vi "SetCaptureFrames.vi"(8 "error in (no error)":errorcluster, 10 "Setting.FramesToCapture":i32, 11 "Camera_Prime95B in":refnum<class "Camera_Prime95B.lvclass">) -> (0 "error out":errorcluster, 3 "Camera_Prime95B out":refnum<class "Camera_Prime95B.lvclass">)   [LabVIEW 2020, in "Camera_Prime95B.lvlib" / "Camera_Prime95B.lvclass"]
uses:
  Camera_Prime95B.lvclass
  Camera_Prime95B.lvclass/Camera_Prime95B.ctl
  E:/Development/DevHardSoftware/MMicroscopyAF/Model/Real Hardware/Camera_Prime95B/Camera_Prime95B/Dependencies/PVCamNET.dll
  Dependencies/PVCamNET.dll
  HAL Layer/Component/Camera/Camera/Camera.lvclass
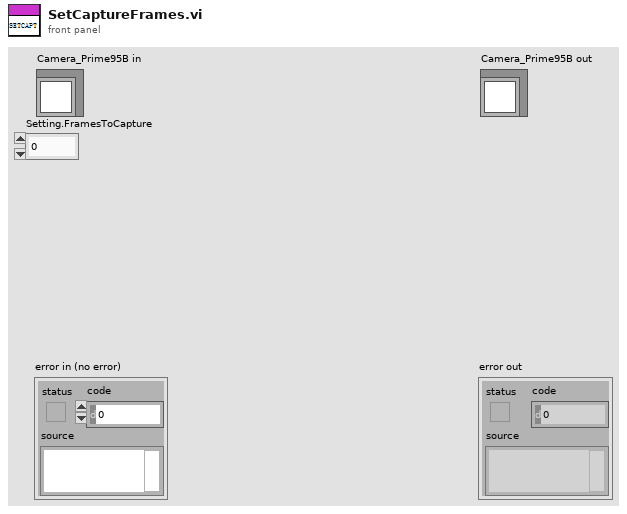
[diagram p1: front panel]
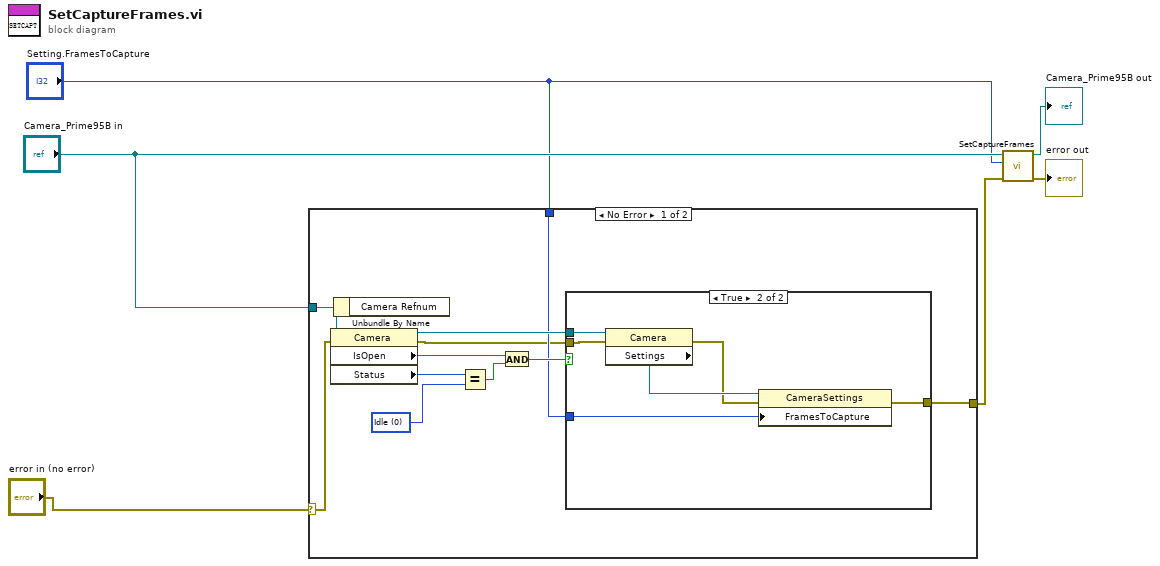
[diagram p0: block diagram]
diagram:
  n1 = case shown="No Error" "error in (no error)" {
    selector: "error in (no error)" -> [w7 w26]
    tunnel: [w9 w26] -> w2
    tunnel: "Camera_Prime95B in" -> [w18 _]
    tunnel: "Setting.FramesToCapture" -> [w10 _]
    frame No Error {
      w16 = 0 items=["Idle", "Capturing"] ("Status")
      n2 = Unbundle By Name(w18) -> ("Camera Refnum"=w15:refnum<k24>)
      n3 = property class="Camera"(reference=w15, error in=w7) -> (reference out=w11:refnum<k24>, error out=w8:errorcluster, "IsOpen"=w13:bool, "Status"=w17:i32)
      n4 = Equal?(x=w17, y=w16) -> (x = y?=w14:bool)
      n5 = And(x=w13, y=w14) -> (x .and. y?=w12:bool)
      n6 = case shown="True" w12 {
        tunnel: [w19 w25] -> w9
        tunnel: w11 -> [_ w22]
        tunnel: w10 -> [_ w21]
        tunnel: w8 -> [w19 w20]
        frame False {
        }
        frame True {
          n7 = property class="Camera"(reference=w22, error in=w20) -> (error out=w23:errorcluster, "Settings"=w24:refnum<k24>)  [unwired: 1 out]
          n8 = property class="CameraSettings"(reference=w24, error in=w23, "FramesToCapture"=w21) -> (error out=w25:errorcluster)  [unwired: 1 out]
        }
      }
    }
    frame Error {
    }
  }
  n9 = call-parent "SetCaptureFrames.vi"("error in (no error)"=w2, "Setting.FramesToCapture"="Setting.FramesToCapture", "Camera in"="Camera_Prime95B in") -> ("error out"=→"error out":errorcluster, "Camera out"=→"Camera_Prime95B out":refnum<class "Camera_Prime95B.lvclass">)  [unwired: 7 in]
